vi "AB_ProgressBar_Fire_New_Job.vi"(8 "error in (no error)":errorcluster, 9 "#ofItems":i32, 10 "Label":string, 11 "progressBarEvents in":T1) -> (0 "error out":errorcluster, 3 "progressBarEvents out":T1)   [LabVIEW 2020]
uses:
  <resource>/Framework/Providers/Common/provcom_ProgressBar_Events.ctl
  <resource>/Framework/Providers/API/mxLvBuildError.ctl
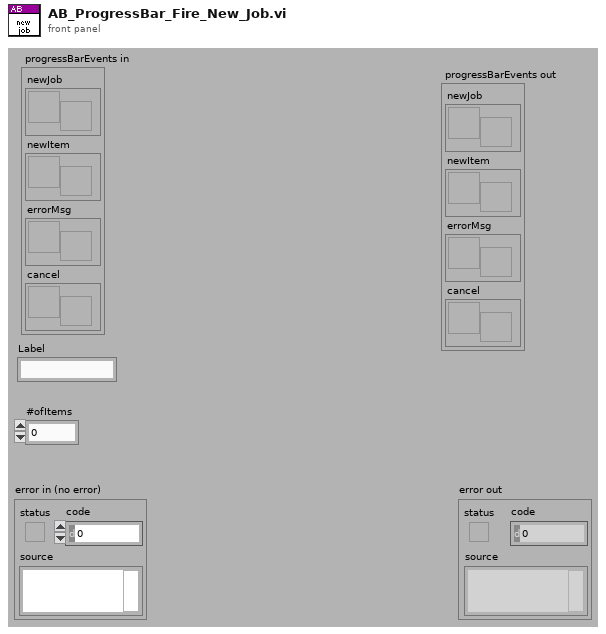
[diagram p1: front panel]
types:
  T1 = typedef "provcom_ProgressBar_Events.ctl" = cluster{"newJob":refnum<user-event>, "newItem":refnum<user-event>, "errorMsg":T2, "cancel":refnum<user-event>}
  T2 = typedef "mxLvBuildError.ctl" = refnum<user-event>
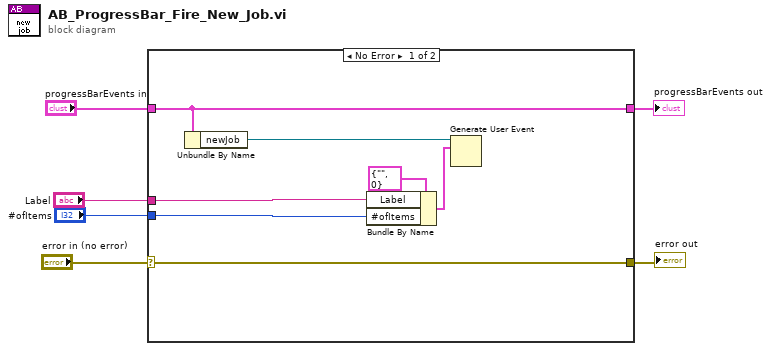
[diagram p0: block diagram]
diagram:
  n1 = case shown="No Error" "error in (no error)" {
    selector: "error in (no error)" -> [w13 w15]
    tunnel: [w13 w15] -> w5
    tunnel: [w10 w14] -> w3
    tunnel: "progressBarEvents in" -> [w10 w14]
    tunnel: "#ofItems" -> [w8 _]
    tunnel: "Label" -> [w7 _]
    frame No Error {
      n2 = Unbundle By Name(w10) -> ("newJob"=w9:refnum<user-event>)
      n3 = Bundle By Name(cluster=cluster{"Label":string, "#ofItems":i32} {"Label"="", "#ofItems"=0} ("event data"), "Label"=w7, "#ofItems"=w8) -> (w11:cluster{"Label":string, "#ofItems":i32})
      n4 = Generate User Event(user event=w9, event data cluster=w11) -> ()  [unwired: 2 in, 2 out]
    }
    frame Error {
    }
  }
  "error out" <- w5
  "progressBarEvents out" <- w3
